vi "Priority.vi"(8 "error in (no error)":errorcluster, 11 "ControllerIndexedPathParams Handler in":refnum<class "ControllerIndexedPathParams Handler.lvclass">) -> (0 "error out":errorcluster, 2 "Priority":u16, 3 "ControllerIndexedPathParams Handler out":refnum<class "ControllerIndexedPathParams Handler.lvclass">)   [LabVIEW 2020]
uses:
  ControllerIndexedPathParams Handler.lvclass
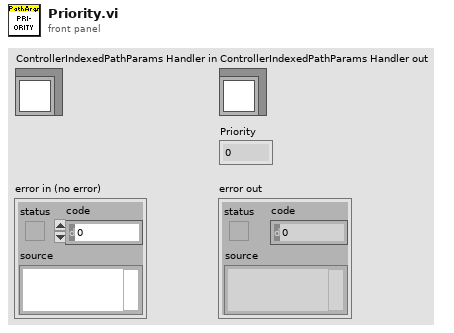
[diagram p1: front panel]
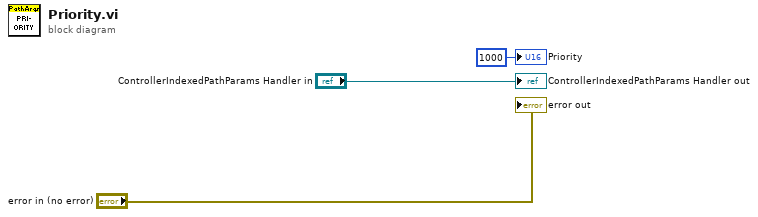
[diagram p0: block diagram]
diagram:
  "error out" <- "error in (no error)"
  "ControllerIndexedPathParams Handler out" <- "ControllerIndexedPathParams Handler in"
  "Priority" <- u16 1000 ("Priority")
